vi "Function Decomposition.VI"(0 "function string":string, 1 "error in (no error)":errorcluster) -> (2 "function text":string, 3 "function brackets":string, 4 "rest":string, 5 "error out":errorcluster)   [LabVIEW 2017, in "NI_Gmath.lvlib"]
uses:
  <vilib>/gmath/NI_Gmath.lvlib
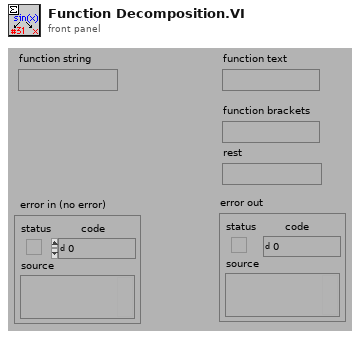
[diagram p1: front panel]
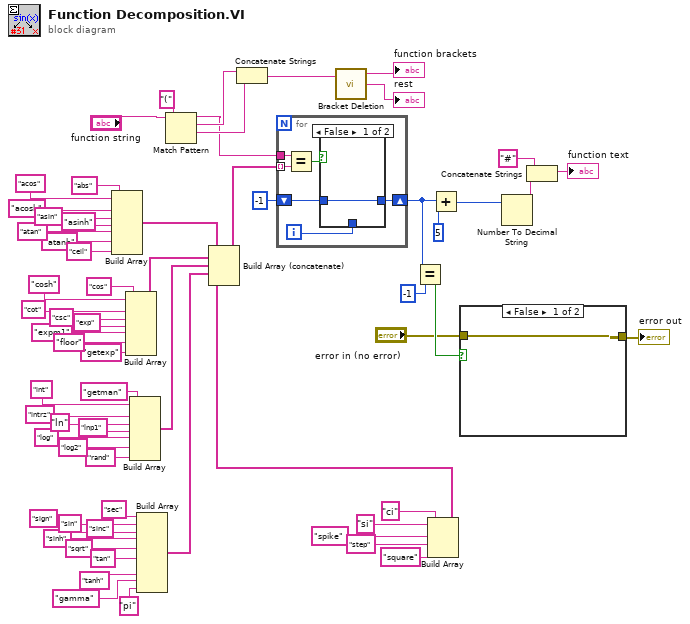
[diagram p0: block diagram]
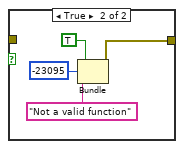
[diagram p2: hidden frame]
diagram:
  n1 = Build Array("abs", "acos", "acosh", "asin", "asinh", "atan", "atanh", "ceil") -> (w19:string[])
  n2 = Build Array("cos", "cosh", "cot", "csc", "exp", "expm1", "floor", "getexp") -> (w18:string[])
  n3 = Build Array("getman", "int", "intrz", "ln", "lnp1", "log", "log2", "rand") -> (w17:string[])
  n4 = Build Array("sec", "sign", "sin", "sinc", "sinh", "sqrt", "tan", "tanh", "gamma", "pi") -> (w16:string[])
  n5 = Match Pattern(string="function string", regular expression="(") -> (before substring=w49:string, match substring=w58:string, after substring=w57:string)  [unwired: 1 in, 1 out]
  n6 = Concatenate Strings(w58, w57) -> (w56:string)
  n7 = call <vilib>:"Bracket Deletion.vi"("string input with brackets"=w56) -> ("string output balanced"=→"function brackets":string, "string output rest"=→"rest":string)  [unwired: 1 in, 1 out]
  n8 = Build Array("ci", "si", "spike", "step", "square") -> (w12:string[])
  n9 = Build Array (concatenate)(w19, w18, w17, w16, w12) -> (w15:string[])
  n10 = for {
    tunnel: w49 -> [w70]
    tunnel: w15 -> [w69] mode=indexing
    shift-right: [w67] -> w6
    shift-left: -1 -> [w68]
    i -> [w65]
    n11 = Equal?(x=w70, y=w69) -> (x = y?=w66:bool)
    n12 = case shown="False" w66 {
      tunnel: w68 -> [w71 _]
      tunnel: [w71 w72] -> w67
      tunnel: w65 -> [_ w72]
      frame False {
      }
      frame True {
      }
    }
  }
  n13 = Equal?(x=w6, y=-1) -> (x = y?=w4:bool)
  n14 = Add(x=w6, y=5) -> (x+y=w52:i32)
  n15 = case shown="False" w4 {
    tunnel: "error in (no error)" -> [w73 _]
    tunnel: [w73 w77] -> w2
    frame False {
    }
    frame True {
      n16 = Bundle(TRUE, -23095, "Not a valid function") -> (w77:errorcluster)  [unwired: 1 in]
    }
  }
  "error out" <- w2
  n17 = Number To Decimal String(number=w52) -> (decimal integer string=w51:string)  [unwired: 1 in]
  n18 = Concatenate Strings("#", w51) -> (→"function text":string)
